vi "Actor Last Ack.vi"(9 "Nest Error":errorcluster, 10 "Nest Actor":refnum<class "Actor.lvclass">, 11 "Actor Last Ack Msg Strategy in":refnum<class "Actor Last Ack Msg Strategy.lvclass">) -> (0 "error out":errorcluster, 3 "Actor Last Ack Msg Strategy out":refnum<class "Actor Last Ack Msg Strategy.lvclass">)   [LabVIEW 2021, in "Actor Last Ack.lvlib" / "Actor Last Ack Msg Strategy.lvclass"]
uses:
  Actor Last Ack Msg Strategy.lvclass
  LVCAM/Actor/Actor.lvclass
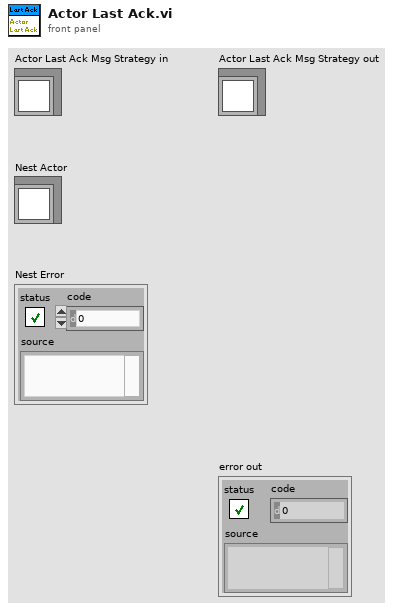
[diagram p1: front panel]
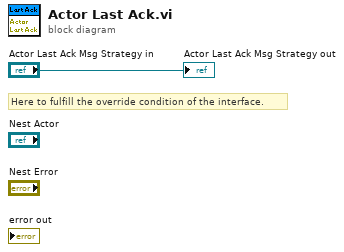
[diagram p0: block diagram]
diagram:
  # "Here to fulfill the override condition of the interface."
  "Actor Last Ack Msg Strategy out" <- "Actor Last Ack Msg Strategy in"
